vi "PS_Plasma_Ball.vi"(11 "On/Off":bool) -> (0 "error out":errorcluster)   [LabVIEW 2011]
uses:
  <vilib>/DAQmx/write.llb/DAQmx Write (Digital Bool 1Line 1Point).vi
  PS_Global.vi
  <vilib>/DAQmx/create/channels.llb/DAQmx Create Channel (DO-Digital Output).vi
  <vilib>/DAQmx/miscellaneous.llb/DAQmx Fill In Error Info.vi
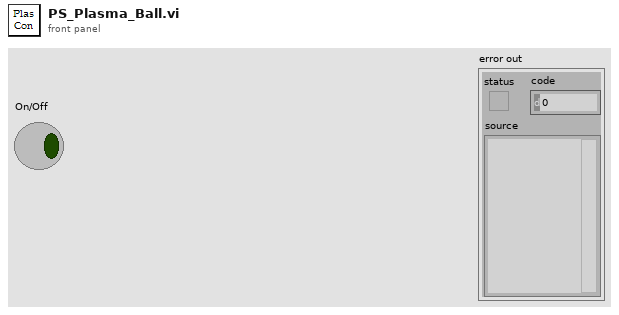
[diagram p1: front panel]
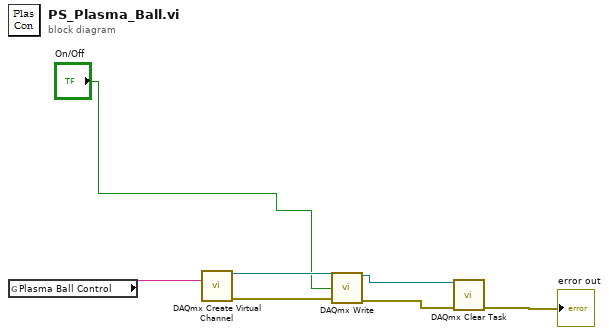
[diagram p0: block diagram]
diagram:
  n1 = global read "PS_Global.vi" "Plasma Ball Control"() -> (w7:tag)
  n2 = call-poly <vilib>:"DAQmx Create Virtual Channel.vi"("lines"=w7) -> ("task out"=w6:refnum<k21>, "error out"=w4:errorcluster)  [unwired: 13 in]
  n3 = call-poly <vilib>:"DAQmx Write.vi"("task/channels in"=w6, "data"="On/Off", "error in"=w4) -> ("task out"=w3:refnum<k21>, "error out"=w2:errorcluster)  [unwired: 10 in, 1 out]
  n4 = call <vilib>:"DAQmx Clear Task.vi"("task in"=w3, "error in"=w2) -> ("error out"=→"error out":errorcluster)  [unwired: 13 in]
